vi "mainSolve.vi"() -> ()   [LabVIEW 2019]
uses:
  deftype controle 3.ctl
panel:
  out "Commands to Execute 5":string[](array[string])
  out "RubixTab patron":string[][](array[string])
  out "RubixTab image":string[][](array[string])
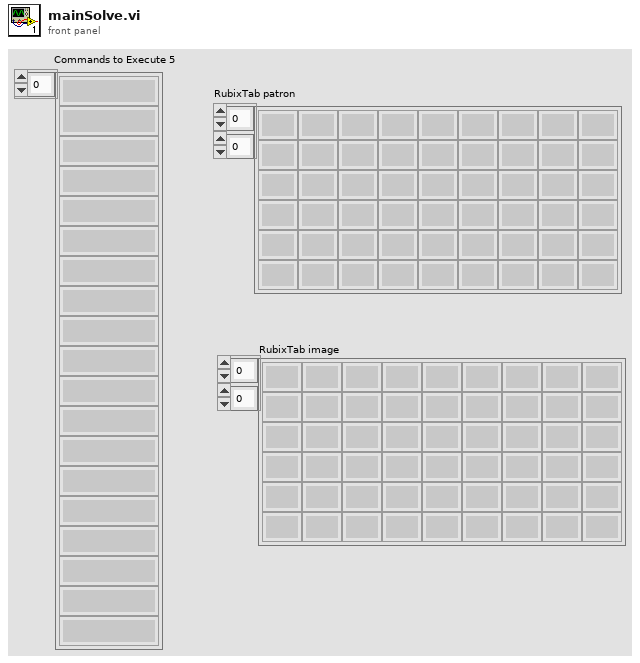
[diagram p1: front panel]
types:
  T1 = typedef "deftype controle 3.ctl" = enum16{"Traitement Image", "control face number ", "PatronCube ", "solution patron corrigé", "solution", "Fin"}
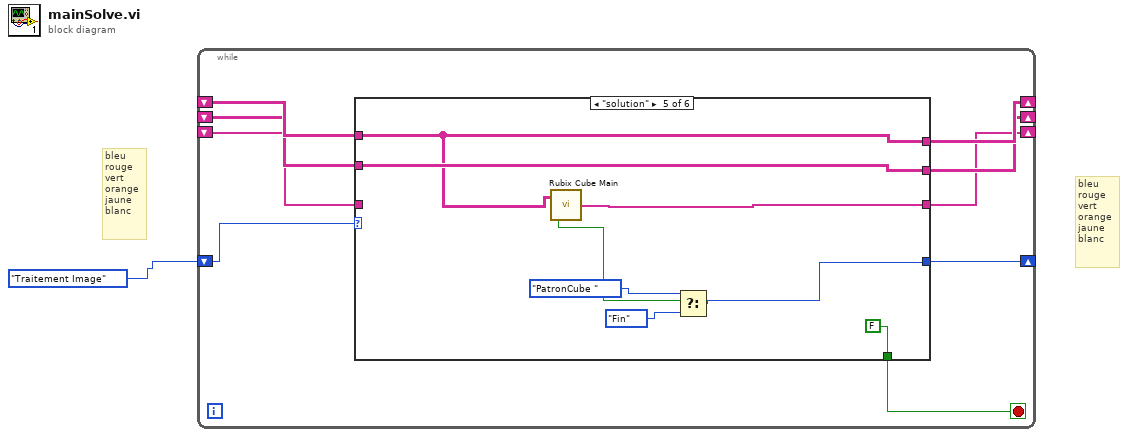
[diagram p0: block diagram]
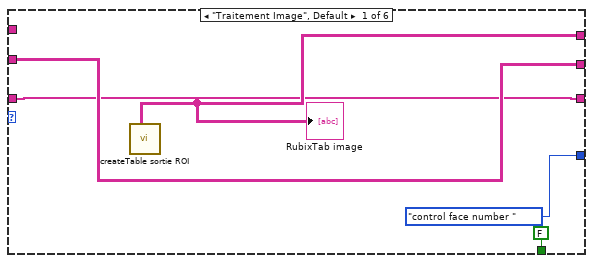
[diagram p2: hidden frame]
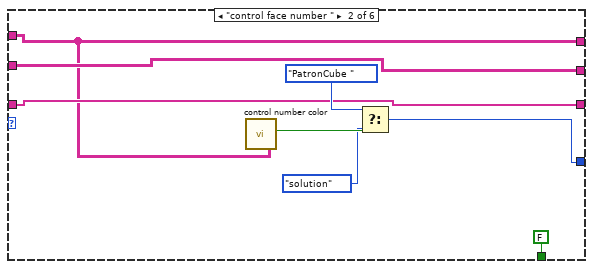
[diagram p3: hidden frame]
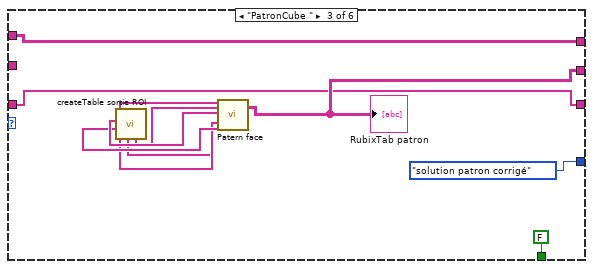
[diagram p4: hidden frame]
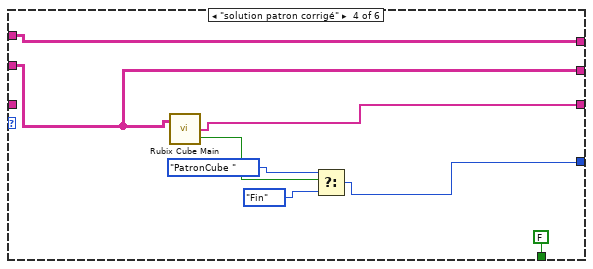
[diagram p5: hidden frame]
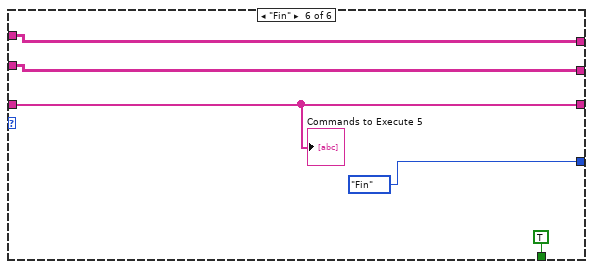
[diagram p6: hidden frame]
diagram:
  # "bleu\nrouge\nvert\norange \njaune \nblanc"
  # "bleu\nrouge\nvert\norange \njaune \nblanc"
  n1 = while {
    shift-right: [w5] -> _
    shift-left: deftype_controle_3."Traitement Image" -> [w10]
    shift-right: [w9] -> _
    shift-left: _ -> [w8]
    shift-right: [w7] -> _
    shift-left: _ -> [w6]
    shift-right: [w3] -> _
    shift-left: _ -> [w2]
    stop <- w4 stop-if-true
    n2 = case shown="\"solution\"" w10 {
      tunnel: [w15 w16 w26 w42 w46 w55] -> w9
      tunnel: w8 -> [_ w16 w26 w42 w46 w55]
      tunnel: [w14 w19 w27 w40 w50 w54] -> w7
      tunnel: w6 -> [w14 w19 _ w40 w50 w54]
      tunnel: [deftype_controle_3."control face number " w22 deftype_controle_3."solution patron corrigé" w35 w43 deftype_controle_3."Fin"] -> w5
      tunnel: [FALSE FALSE FALSE FALSE FALSE TRUE] -> w4
      tunnel: [w11 w17 w24 w39 w45 w51] -> w3
      tunnel: w2 -> [w11 w17 w24 _ _ w51]
      frame "Traitement Image", Default {
        n3 = call "createTable sortie ROI.vi"() -> ("RubixTab solver"=w15:string[][])  [unwired: 5 in, 6 out]
        "RubixTab image" <- w15
      }
      frame "control face number " {
        n4 = call "control number color.vi"("arrivée traitement"=w16) -> ("True"=w23:bool)  [unwired: 7 out]
        n5 = Select(t=deftype_controle_3."PatronCube ", s=w23, f=deftype_controle_3."solution") -> (s? t:f=w22:T1)
      }
      frame "PatronCube " {
        n6 = call "createTable sortie ROI.vi"() -> ("Face 4 blanche"=w28:string[], "Face 2 jaune"=w29:string[], "Face 3 orange"=w30:string[], "Face 6 verte"=w31:string[], "Face 1 rouge"=w32:string[], "Face 5 bleu"=w33:string[])  [unwired: 5 in, 1 out]
        n7 = call "Patern face.vi"("bleue"=w33, "blanc"=w28, "Rouge"=w32, "Vert"=w31, "Orange"=w30, "Jaune"=w29) -> ("RubixTab solver"=w27:string[][])  [unwired: 13 in]
        "RubixTab patron" <- w27
      }
      frame "solution patron corrigé" {
        n8 = call "Rubix Cube Main.vi"("RubixTab patron"=w40) -> ("Commands to Execute"=w39:string[], "Boolean"=w38:bool)
        n9 = Select(t=deftype_controle_3."PatronCube ", s=w38, f=deftype_controle_3."Fin") -> (s? t:f=w35:T1)
      }
      frame "solution" {
        n10 = call "Rubix Cube Main.vi"("RubixTab patron"=w46) -> ("Commands to Execute"=w45:string[], "Boolean"=w44:bool)
        n11 = Select(t=deftype_controle_3."PatronCube ", s=w44, f=deftype_controle_3."Fin") -> (s? t:f=w43:T1)
      }
      frame "Fin" {
        "Commands to Execute 5" <- w51
      }
    }
  }
